vi "Write.vi"(8 "error in (no error)":errorcluster, 10 "Write Data":variant, 11 "Modbus PLC in":refnum<class "Modbus PLC.lvclass">) -> (0 "error out":errorcluster, 3 "Modbus PLC out":refnum<class "Modbus PLC.lvclass">)   [LabVIEW 2023, in "Modbus PLC.lvlib" / "Modbus PLC.lvclass"]
uses:
  Modbus PLC.lvclass
  Commands.ctl
  Modbus PLC.lvclass/Modbus PLC.ctl
  <vilib>/NI/Modbus Library/API/Master/Modbus Master.lvclass
panel:
  in  "CMD":T1 {"Mix_CMD" items=["Мешалка движение вперёд"=1, "Мешалка движение назад"=2, "Мешалка стоп"=9]; "Termex_CMD" items=["Термостат старт"=1, "Термостат стоп"=9]; "Rotate_CMD" items=["Качалка Дом"=1, "Качалка Режим Авто - Старт"=2, "Качалка Режим Ручной - Старт"=3, "Качалка Стоп"=9]}
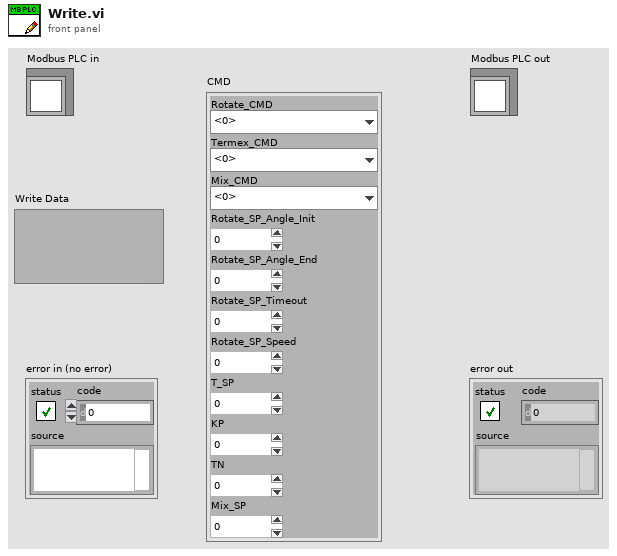
[diagram p1: front panel]
types:
  T1 = typedef "Modbus PLC.lvlib/Modbus PLC.lvclass/Commands.ctl" = cluster{"Rotate_CMD":u16, "Termex_CMD":u16, "Mix_CMD":u16, "Rotate_SP_Angle_Init":u16, "Rotate_SP_Angle_End":u16, "Rotate_SP_Timeout":u16, "Rotate_SP_Speed":u16, "T_SP":sgl, "KP":sgl, "TN":sgl, "Mix_SP":u16}
  T2 = typedef "Modbus PLC.lvlib/Modbus PLC.lvclass/Input Map.ctl" = map{string, cluster{"Address":i32, "Data Type":enum16{"Int", "Float"}, "Reg Type":enum16{"Holding", "Input", "Coil"}}}
  T3 = cluster{"Address":i32, "Data Type":enum16{"Int", "Float"}, "Reg Type":enum16{"Holding", "Input", "Coil"}}
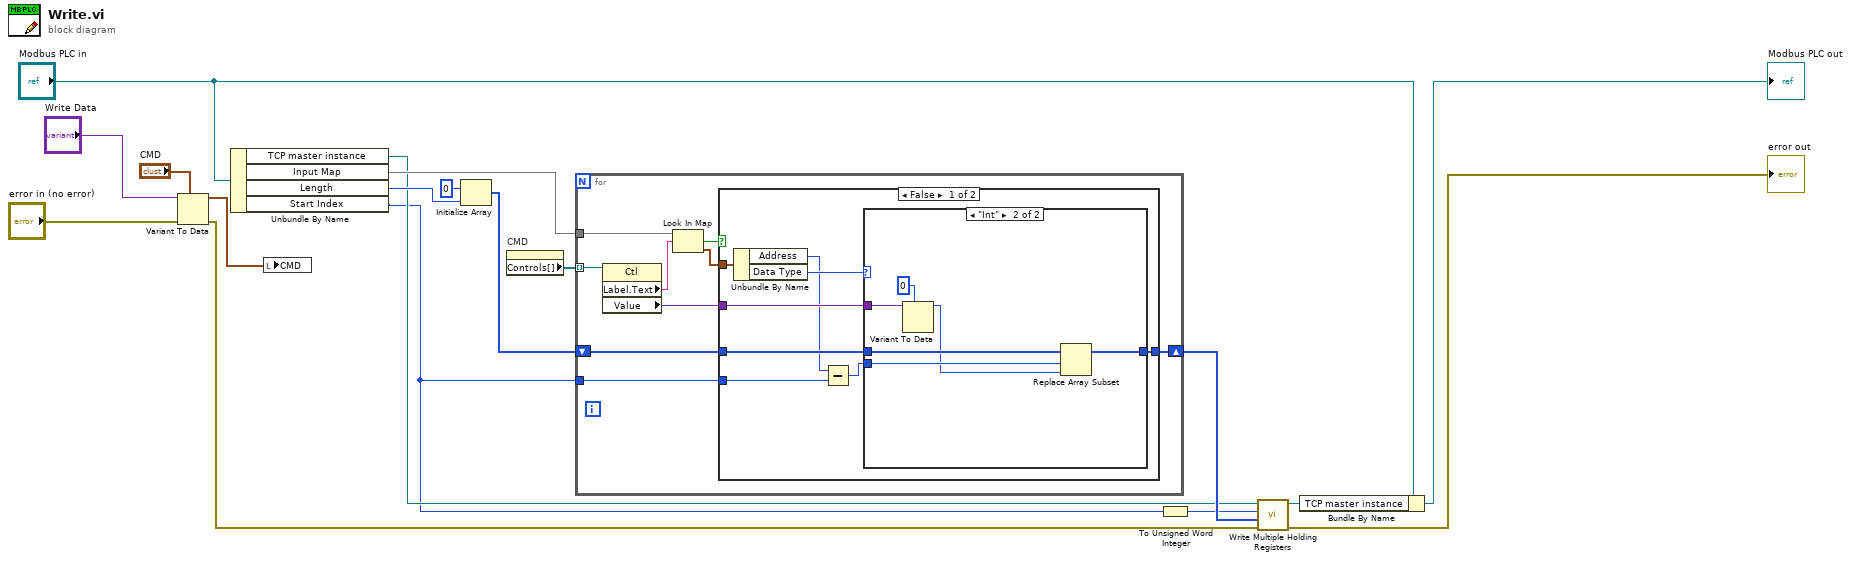
[diagram p0: block diagram]
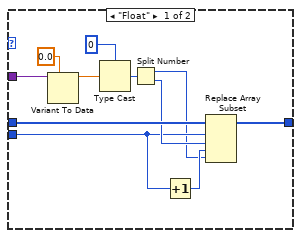
[diagram p2: hidden frame]
diagram:
  n1 = Variant To Data(error in="error in (no error)", type="CMD", Variant="Write Data") -> (data=w3:T1, error out=w8:errorcluster)
  n2 = Unbundle By Name("Modbus PLC in") -> ("TCP master instance"=w9:refnum<class "Modbus Master.lvclass">, "Input Map"=w15:T2, "Length"=w12:u16, "Start Index"=w4:u16)
  n3 = local write "CMD"(w3) -> ()
  n4 = Initialize Array(u16 0, w12) -> (w11:u16[])
  n5 = property on="CMD" class="Clust (strict)"() -> ("Controls[]"=w14:refnum<vi>[])  [unwired: 2 in, 2 out]
  n6 = for {
    tunnel: w15 -> [w27]
    tunnel: w14 -> [w26] mode=indexing
    shift-right: [w20] -> w10
    shift-left: w11 -> [w21]
    tunnel: w4 -> [w19]
    n7 = property class="Ctl"(reference=w26) -> ("Label.Text"=w25:string, "Value"=w22:variant)  [unwired: 1 in, 2 out]
    n8 = Look In Map(map=w27, key=w25) -> (key not found?=w24:bool, value=w23:T3)  [unwired: 1 in]
    n9 = case shown="False" w24 {
      tunnel: w23 -> [w35 _]
      tunnel: w22 -> [w33 _]
      tunnel: w21 -> [w32 w53]
      tunnel: [w31 w53] -> w20
      tunnel: w19 -> [w29 _]
      frame False {
        n10 = Unbundle By Name(w35) -> ("Address"=w28:i32, "Data Type"=w34:enum16{"Int", "Float"})
        n11 = Subtract(x=w28, y=w29) -> (x-y=w30:i32)
        n12 = case shown="\"Int\"" w34 {
          tunnel: w33 -> [w46 w52]
          tunnel: w32 -> [w41 w50]
          tunnel: w30 -> [w38 w49]
          tunnel: [w36 w48] -> w31
          frame "Float" {
            n13 = Variant To Data(type=sgl 0.0, Variant=w46) -> (data=w44:sgl)  [unwired: 1 in, 1 out]
            n14 = Type Cast(type=u32 0, x=w44) -> (*(type *) &x=w42:u32)
            n15 = Split Number(x=w42) -> (hi(x)=w37:u16, lo(x)=w40:u16)
            n16 = Increment(x=w38) -> (x+1=w39:i32)
            n17 = Replace Array Subset(array=w41, new element #1=w40, index #1=w38, new element #2=w37, index #2=w39) -> (w36:u16[])
          }
          frame "Int" {
            n18 = Variant To Data(type=u16 0, Variant=w52) -> (data=w47:u16)  [unwired: 1 in, 1 out]
            n19 = Replace Array Subset(array=w50, new element=w47, index=w49) -> (w48:u16[])
          }
        }
      }
      frame True {
      }
    }
  }
  n20 = To Unsigned Word Integer(number=w4) -> (unsigned 16bit integer=w5:u16)
  n21 = call-dynamic "Write Multiple Holding Registers.vi"("error in"=w8, "registers to write"=w10, "starting address"=w5, "Modbus master in"=w9) -> ("error out"=→"error out":errorcluster, "Modbus master out"=w6:refnum<class "Modbus Master.lvclass">)  [unwired: 6 in]
  n22 = Bundle By Name(cluster="Modbus PLC in", "TCP master instance"=w6) -> (→"Modbus PLC out":refnum<class "Modbus PLC.lvclass">)
